vi "hidSPD Write Multi Reports.vi"(8 "error in (no error)":errorcluster, 10 "hidSPD Controller Setup reportd":T1[](array[typedef]) {"HV_bias" format="%#_6p, V"; "TSet" format="%#_6p, DegC"}, 11 "spdDevSessions in":T2[](array[typedef]) {"hidSPD.Controller"."HV_bias" format="%#_6p, V"; "hidSPD.Controller"."TSet" format="%#_6p, DegC"}) -> (0 "error out":errorcluster, 3 "spdDevSessions out":T2[](array[typedef]) {"hidSPD.Controller"."HV_bias" format="%#_6p, V"; "hidSPD.Controller"."TSet" format="%#_6p, DegC"})   [LabVIEW 2018, in "hidSPDLibForLabView.lvlib"]
uses:
  hidSPDLibForLabView.lvlib
  hidSPD Controls/hidSPD Device Session.ctl
  hidSPD Controls/hidSPD Controller.ctl
  hidSPD Controls/hidSPD Controller Setup Report.ctl
  hidSPD Write Report/hidSPD Setup Controller.vi
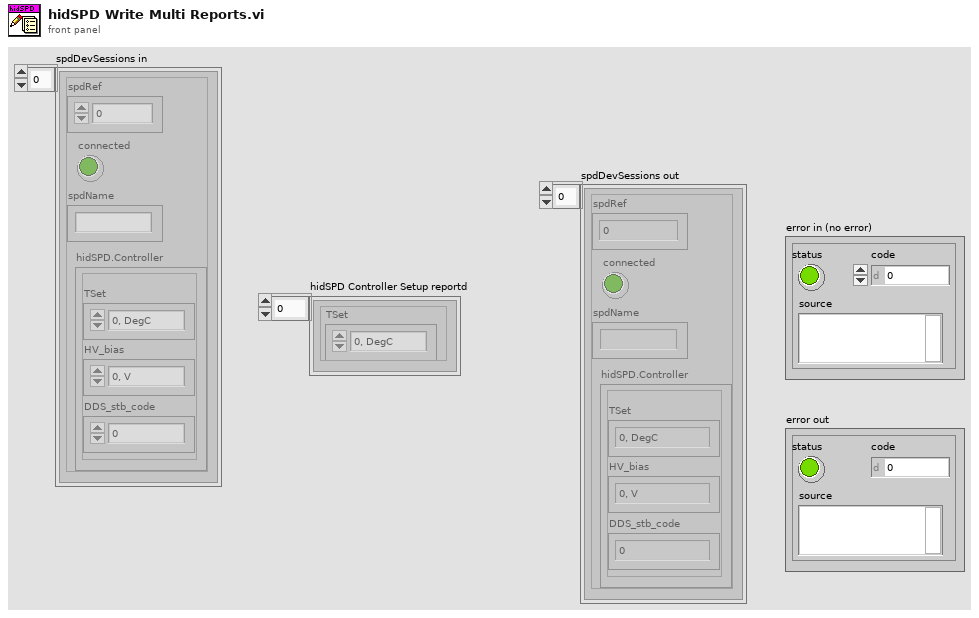
[diagram p1: front panel]
types:
  T1 = typedef "hidSPDLibForLabView.lvlib/hidSPD Controller Setup Report.ctl" = cluster{"TSet":sgl, "HV_bias":sgl, "DDS_stb_code":u16, "SPD_reset":u16, "MCU_reset":u16}
  T2 = typedef "hidSPDLibForLabView.lvlib/hidSPD Device Session.ctl" = cluster{"spdRef":u64, "connected":bool, "spdName":string, "hidSPD.Controller":T3}
  T3 = typedef "hidSPDLibForLabView.lvlib/hidSPD Controller.ctl" = cluster{"TSet":sgl, "HV_bias":sgl, "DDS_stb_code":u16}
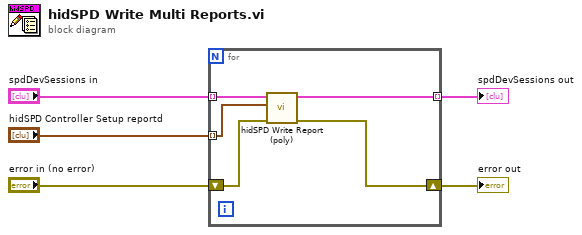
[diagram p0: block diagram]
diagram:
  n1 = for {
    tunnel: "spdDevSessions in" -> [w10] mode=indexing
    shift-right: [w8] -> w3
    shift-left: "error in (no error)" -> [w7]
    tunnel: [w9] -> w2 mode=indexing
    tunnel: "hidSPD Controller Setup reportd" -> [w6] mode=indexing
    n2 = call-poly "hidSPD Write Report (poly).vi"("error in (no error)"=w7, "hidSPD Controller Setup report"=w6, "spdDevSession in"=w10) -> ("error out"=w8:errorcluster, "spdDevSession out"=w9:T2)  [unwired: 7 in]
  }
  "error out" <- w3
  "spdDevSessions out" <- w2
